vi "Set Values.vi"(6 "Target":dbl, 8 "error in (no error)":errorcluster, 9 "Step Time":dbl, 10 "Step Temp":dbl, 11 "Rate Step in":refnum<class "Rate Step.lvclass">) -> (0 "error out":errorcluster, 3 "Rate Step out":refnum<class "Rate Step.lvclass">)   [LabVIEW 2018, in "Temp Recipe.lvlib" / "Rate Step.lvclass"]
uses:
  Rate Step.lvclass
  C:/dev/source/Systems/NI Week/Temperature Recipe/Temp Recipe/Recipe Step/Recipe Step.lvclass
  Rate Step.lvclass/Rate Step.ctl
  Recipe Step/Recipe Step.lvclass
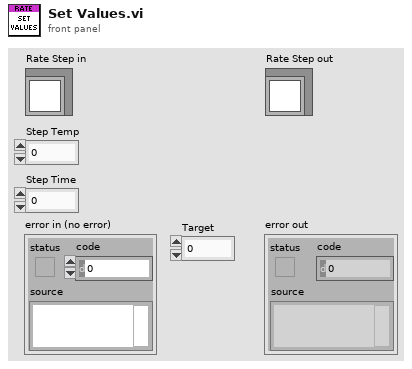
[diagram p1: front panel]
types:
  T1 = typedef "Temp Recipe.lvlib/Rate Step.lvclass/Ref Data.ctl" = cluster{"Step Temp":dbl, "Step Time":dbl, "Target":dbl}
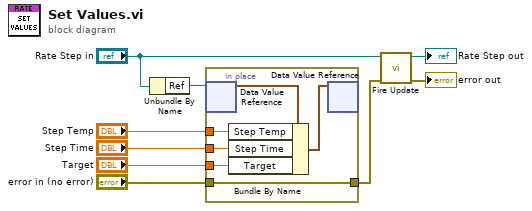
[diagram p0: block diagram]
diagram:
  n1 = Unbundle By Name("Rate Step in") -> ("Ref"=w9:refnum<data-value>)
  n2 = in-place {
    in-place-border: "Step Temp" -> [w13]
    in-place-border: "Step Time" -> [w12]
    in-place-border: "Target" -> [w11]
    in-place-border: "error in (no error)" -> [w10]
    in-place-border: [w10] -> w3
    n3 = in-place-dvr #1(w9) -> (w15:T1)  [unwired: 1 out]
    n4 = Bundle By Name(cluster=w15, "Step Temp"=w13, "Step Time"=w12, "Target"=w11) -> (w14:T1)
    n5 = in-place-dvr #1(w14) -> ()  [unwired: 2 out]
  }
  n6 = call "Fire Update.vi"("error in (no error)"=w3, "Recipe Step in"="Rate Step in") -> ("error out"=→"error out":errorcluster, "Recipe Step out"=→"Rate Step out":refnum<class "Rate Step.lvclass">)  [unwired: 8 in]
